vi "Destroy.vi"(8 "error in":errorcluster, 11 "measurement context in":refnum<class "Measure Call Context.lvclass">) -> (0 "error out":errorcluster)   [LabVIEW 2020, in "Measurement Plugin Measurement Server.lvlib" / "Measure Call Context.lvclass"]
uses:
  Measure Call Context.lvclass
  Measure Call Context.lvclass/Measure Call Context.ctl
  Measurement Plugin Session Management Client/RPC Messages/ni_measurementlink_sessionmanagement_v1_UnreserveSessionsRequest.ctl
  Measurement Plugin Session Management Client/RPC Messages/ni_measurementlink_sessionmanagement_v1_SessionInformation.ctl
  Measurement Plugin Session Management Client/RPC Messages/nidevice_grpc_Session.ctl
  Measurement Plugin Session Management Client/RPC Messages/ni_measurementlink_sessionmanagement_v1_ChannelMapping.ctl
  Measurement Plugin Session Management Client/Measurement Plugin Session Management Client.lvlib
  Measurement Plugin Session Management V1/Session Reservation/Session Reservation.lvclass
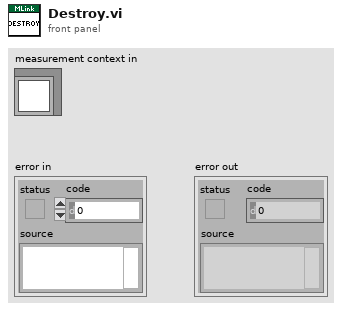
[diagram p1: front panel]
types:
  T1 = typedef "Measurement Plugin Session Management Client.lvlib/ni_measurementlink_sessionmanagement_v1_UnreserveSessionsRequest.ctl" = cluster{"sessions":T2[]}
  T2 = typedef "Measurement Plugin Session Management Client.lvlib/ni_measurementlink_sessionmanagement_v1_SessionInformation.ctl" = cluster{"session":T3, "resource_name":string, "channel_list":string, "instrument_type_id":string, "session_exists":bool, "channel_mappings":T4[]}
  T3 = typedef "Measurement Plugin Session Management Client.lvlib/nidevice_grpc_Session.ctl" = cluster{"name":string}
  T4 = typedef "Measurement Plugin Session Management Client.lvlib/ni_measurementlink_sessionmanagement_v1_ChannelMapping.ctl" = cluster{"pin_or_relay_name":string, "site":i32, "channel":string, "multiplexer_resource_name":string, "multiplexer_route":string}
  T5 = typedef "Measurement Plugin Measurement Server.lvlib/Measure Call Context.lvclass/Data.ctl" = cluster{"pin map context":T6, "gRPC ID":T7, "measurement service":refnum<class "IMeasurement Service.lvclass">, "measurement plugin service":refnum<class "Measurement Plugin Service.lvclass">, "reserved session infos":set{T8}}
  T6 = typedef "Measurement Plugin Measurement Server.lvlib/Pin Map Context.ctl" = cluster{"pin map id":string, "sites":i32[]}
  T7 = typedef "grpc-lvsupport-release.lvlib/grpcId.ctl" = u64
  T8 = typedef "MeasurementLink Session Management Client.lvlib/ni_measurementlink_sessionmanagement_v1_SessionInformation.ctl" = cluster{"session":T9, "resource_name":string, "channel_list":string, "instrument_type_id":string, "session_exists":bool, "channel_mappings":T10[]}
  T9 = typedef "MeasurementLink Session Management Client.lvlib/nidevice_grpc_Session.ctl" = cluster{"name":string}
  T10 = typedef "MeasurementLink Session Management Client.lvlib/ni_measurementlink_sessionmanagement_v1_ChannelMapping.ctl" = cluster{"pin_or_relay_name":string, "site":i32, "channel":string, "multiplexer_resource_name":string, "multiplexer_route":string}
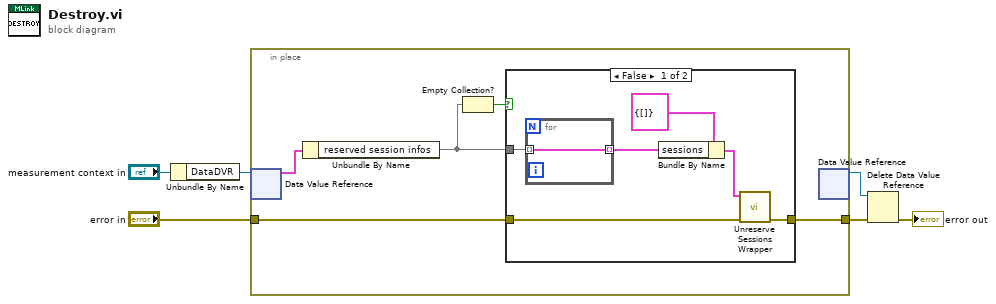
[diagram p0: block diagram]
diagram:
  n1 = Unbundle By Name("measurement context in") -> ("DataDVR"=w5:refnum<data-value>)
  n2 = in-place {
    in-place-border: [w10] -> w2
    in-place-border: "error in" -> [w7]
    n3 = in-place-dvr #1(w5) -> (w11:T5)  [unwired: 1 out]
    n4 = Unbundle By Name(w11) -> ("reserved session infos"=w9:set{T8})
    n5 = Empty Collection?(1:w9) -> (0:w8:bool)
    n6 = case shown="False" w8 {
      tunnel: [w13 w19] -> w10
      tunnel: w9 -> [w15 _]
      tunnel: w7 -> [w12 w19]
      frame False {
        n7 = for {
          tunnel: w15 -> [w18] mode=indexing
          tunnel: [w18] -> w16 mode=indexing
        }
        n8 = Bundle By Name(cluster=T1 {"sessions"=[]} ("Request Data"), "sessions"=w16) -> (w14:T1)
        n9 = call "Unreserve Sessions Wrapper.vi"("error in"=w12, "request data"=w14) -> ("error out"=w13:errorcluster)  [unwired: 8 in, 1 out]
      }
      frame True {
      }
    }
    n10 = in-place-dvr #1() -> (w4:refnum<data-value>)  [unwired: 1 in, 1 out]
  }
  n11 = Delete Data Value Reference(data value reference=w4, error in=w2) -> (error out=→"error out":errorcluster)  [unwired: 1 out]
